vi "Configure Reference Clock.vi"(8 "error in (no error)":errorcluster, 9 "Auto Source (F: Disable)":bool, 10 "Reference Clock Source (0: Internal)":u16(ring) items=["Internal", "External"], 11 "VISA resource name":refnum<visa-resource-name>) -> (0 "error out":errorcluster, 3 "VISA resource name out":refnum<visa-resource-name>)   [LabVIEW 2009, in "Agilent 81150.lvlib"]
doc: "Configures reference clock of the function generator."
uses:
  Agilent 81150.lvlib
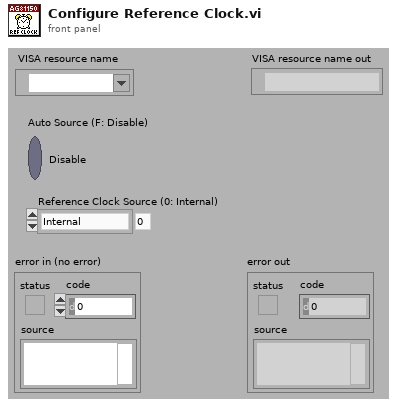
[diagram p1: front panel]
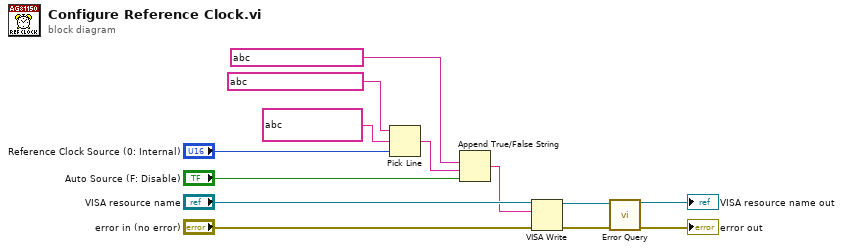
[diagram p0: block diagram]
diagram:
  n1 = Pick Line(string ("")=string ?, multi-line string=string ?, line index="Reference Clock Source (0: Internal)") -> (output string=w2:string)
  n2 = Append True/False String(1:"Auto Source (F: Disable)", 2:w2, 3:string ?) -> (0:w5:string)  [unwired: 1 out]
  n3 = VISA Write(VISA resource name="VISA resource name", write buffer=w5, error in (no error)="error in (no error)") -> (VISA resource name out=w10:refnum<visa-resource-name>, error out=w9:errorcluster)  [unwired: 1 out]
  n4 = call "Error Query.vi"("error in (no error)"=w9, "VISA resource name"=w10) -> ("error out"=→"error out":errorcluster, "VISA resource name out"=→"VISA resource name out":refnum<visa-resource-name>)  [unwired: 8 out]
